vi "Generate Sound - SFP.vi"() -> ()   [LabVIEW 2022 SP3]
uses:
  <vilib>/addons/_NISVFA/_Generation/Signal Generation/SV Signal/sv_System Timing Model.ctl
  <vilib>/addons/_NISVFA/_Generation/Signal Generation/SV Sinusoid/SV Sinusoid.lvclass
  C:/Program Files/NI/LVAddons/nisvt/1/vi.lib/addons/_NISVFA/_Generation/Signal Generation/SV Signal/SV Signal.lvclass
  <vilib>/DAQmx/write.llb/DAQmx Write (Analog Wfm 1Chan NSamp).vi
  <vilib>/DAQmx/create/channels.llb/DAQmx Create Channel (AO-Voltage-Basic).vi
  <vilib>/DAQmx/configure/timing.llb/DAQmx Timing (Sample Clock).vi
  <vilib>/addons/_NISVFA/_Generation/Signal Generation/SV Signal/Write Sample Rate.vi
  <vilib>/addons/_NISVFA/_Generation/Signal Generation/SV Signal/Write System Timing Model.vi
  <vilib>/addons/_NISVFA/_Generation/Signal Generation/SV Signal/Write Ramp Parameters.vi
  <vilib>/addons/_NISVFA/_Generation/Signal Generation/SV Sinusoid/Configure Sine.vi
  <vilib>/DAQmx/miscellaneous.llb/DAQmx Fill In Error Info.vi
  <vilib>/addons/_NISVFA/_Generation/Signal Generation/SV Signal/SV Signal.lvclass
  <resource>/objmgr/daqmx.rc
panel:
  in  "Stop":bool
  in  "output voltage ratio":dbl=0.91 format="%#_g Pa/V"
  in  "amplitude":dbl=94.0 format="%#_g dBSPL"
  in  "output channels":tag="PXI1Slot2/ao0"
  in  "frequency":dbl=1000.0 format="%#_g Hz"
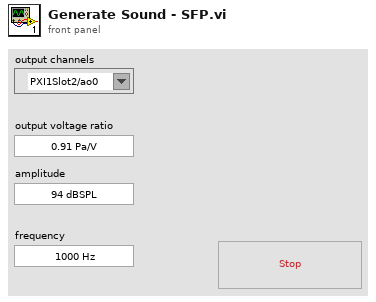
[diagram p1: front panel]
types:
  T1 = typedef "SV Signal.lvclass/sv_System Timing Model.ctl" = i64
  T2 = cluster{"profile":enum16{"Linear", "Half cosine"}, "durations [s]":cluster{"ramp-up":dbl, "transition":dbl, "ramp-down":dbl}}
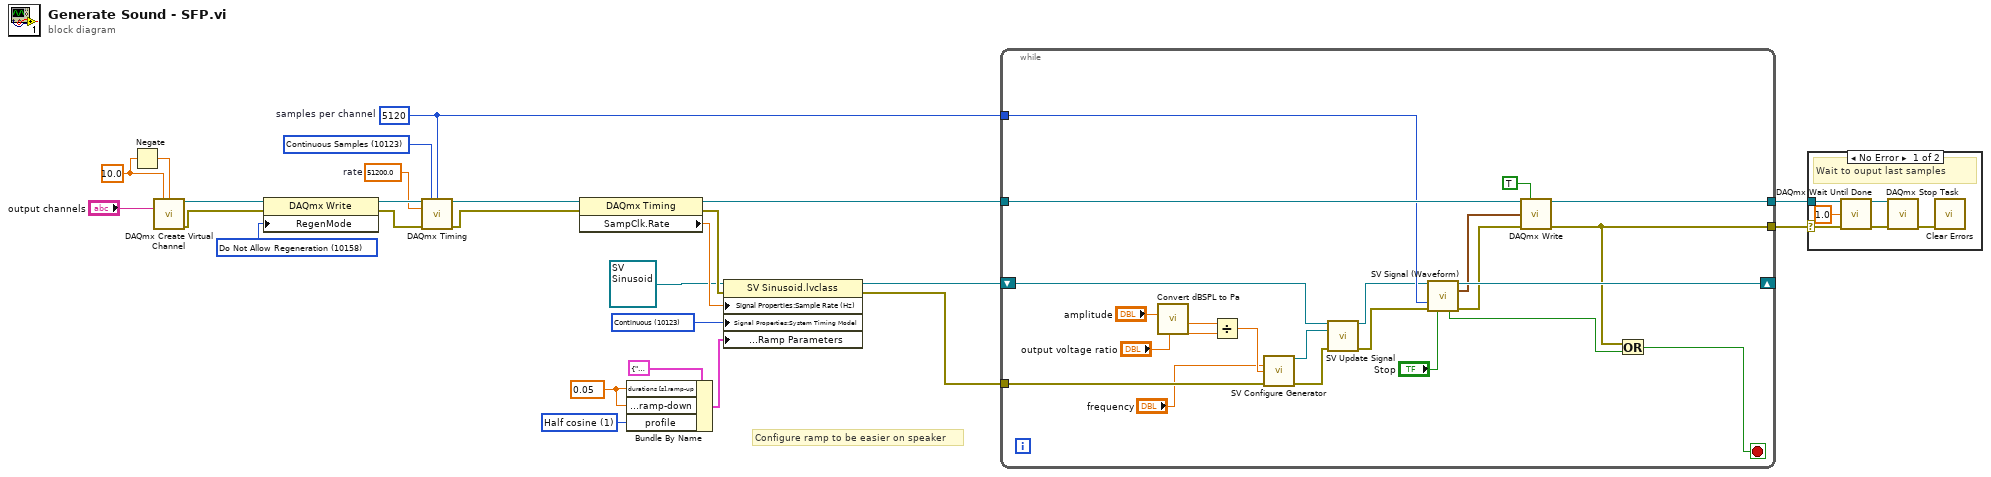
[diagram p0: block diagram]
diagram:
  w25 = 0.05 ("ramp duration")
  w23 = u16 1 items=["Linear", "Half cosine"] ("ramp profile")
  w14 = 10158 items=["Allow Regeneration"=10097, "Do Not Allow Regeneration"=10158] ("RegenMode")
  w17 = 10.0 ("maximum value")
  w6 = 5120  # samples per channel
  w19 = 10123 items=["Finite Samples"=10178, "Continuous Samples"=10123, "Hardware Timed Single Point"=12522] ("sample mode")
  w7 = 51200.0  # rate
  w22 = T1 10123 items=["Finite"=10178, "-"=-1, "Continuous"=10123, "-"=-2, "Settled"=110123, "Averaged"=210123, "Discrete Sweep"=310123, "Continuous Sweep"=410123] ("System Timing Model")
  # "Configure ramp to be easier on speaker"
  n1 = Negate(x=w17) -> (-x=w16:dbl)
  n2 = call-poly <vilib>:"DAQmx Create Virtual Channel.vi"("maximum value"=w17, "minimum value"=w16, "physical channels"="output channels") -> ("task out"=w13:refnum<k21>, "error out"=w11:errorcluster)  [unwired: 11 in]
  n3 = property class="DAQmx Write"(reference=w13, error in=w11, "RegenMode"=w14) -> (reference out=w12:refnum<k21>, error out=w10:errorcluster)
  n4 = call-poly <vilib>:"DAQmx Timing.vi"("task/channels in"=w12, "sample mode"=w19, "samples per channel"=w6, "rate"=w7, "error in"=w10) -> ("task out"=w20:refnum<k21>, "error out"=w18:errorcluster)  [unwired: 9 in]
  n5 = property class="DAQmx Timing"(reference=w20, error in=w18) -> (reference out=w4:refnum<k21>, error out=w8:errorcluster, "SampClk.Rate"=w9:dbl)
  n6 = Bundle By Name(cluster=T2 {"profile"=enum."Linear", "durations [s]"={"ramp-up"=0.0, "transition"=0.0, "ramp-down"=0.0}} ("Ramp Parameters:All Elements"), "durations [s].ramp-up"=w25, "durations [s].ramp-down"=w25, "profile"=w23) -> (w24:T2)
  n7 = property class="SV Sinusoid.lvclass"(reference=refnum<class "SV Sinusoid.lvclass"> refnum, error in=w8, "Signal Properties:Sample Rate (Hz)"=w9, "Signal Properties:System Timing Model"=w22, "Signal Properties:Ramps:Ramp Parameters"=w24) -> (reference out=w2:refnum<class "SV Sinusoid.lvclass">, error out=w3:errorcluster)
  n8 = while {
    shift-right: [w48] -> _
    shift-left: w2 -> [w40]
    tunnel: w6 -> [w42]
    tunnel: w4 -> [w47]
    tunnel: [w46] -> w15
    tunnel: w3 -> [w37]
    tunnel: [w34] -> w5
    stop <- w38 stop-if-true
    n9 = call "Convert dBSPL to Pa.vi"("dB SPL"="amplitude") -> ("Pa pk"=w29:dbl)  [unwired: 9 in, 1 out]
    n10 = Divide(x=w29, y="output voltage ratio") -> (x/y=w31:dbl)
    n11 = call-poly <vilib>:"SV Configure Generator.vi"("frequency (Hz)"="frequency", "amplitude"=w31, "error in (no error)"=w37) -> ("signal configuration"=w41:refnum<class "SV Sinusoid.lvclass">, "error out"=w36:errorcluster)  [unwired: 11 in]
    n12 = call-dynamic "SV Update Signal.vi"("current configuration"=w40, "new configuration"=w41, "error in"=w36) -> ("updated configuration"=w39:refnum<class "SV Sinusoid.lvclass">, "error out"=w35:errorcluster)  [unwired: 11 in]
    n13 = call-dynamic "SV Signal (Waveform).vi"("signal configuration"=w39, "samples"=w42, "error in (no error)"=w35, "stop"="Stop") -> ("signal configuration"=w48:refnum<class "SV Sinusoid.lvclass">, "output waveform"=w43:waveform(dbl), "done"=w33:bool, "error out"=w45:errorcluster)  [unwired: 6 in, 2 out]
    n14 = call-poly <vilib>:"DAQmx Write.vi"("task/channels in"=w47, "auto start"=TRUE, "data"=w43, "error in"=w45) -> ("task out"=w46:refnum<k21>, "error out"=w34:errorcluster)  [unwired: 9 in, 1 out]
    n15 = Or(x=w34, y=w33) -> (x .or. y?=w38:bool)
  }
  n16 = case shown="No Error" w5 {
    selector: w5 -> [w51 _]
    tunnel: w15 -> [w54 _]
    frame No Error {
      # "Wait to ouput last samples"
      n17 = call <vilib>:"DAQmx Wait Until Done.vi"("task/channels in"=w54, "timeout (sec)"=1.0, "error in"=w51) -> ("task out"=w53:refnum<k21>, "error out"=w52:errorcluster)  [unwired: 11 in]
      n18 = call <vilib>:"DAQmx Stop Task.vi"("task/channels in"=w53, "error in"=w52) -> ("error out"=w50:errorcluster)  [unwired: 12 in, 1 out]
      n19 = call <vilib>:"Clear Errors.vi"("error in (no error)"=w50) -> ()  [unwired: 5 in, 2 out]
    }
    frame Error {
      # "Error"
    }
  }
